vi "Complex Spectrum Averaging.vi"(3 "reset averaging (T)":bool=TRUE, 4 "number of averages":u32=10 min=1, 5 "weighting mode":enum16{"Linear", "Exponential"}(ring), 6 "complex spectrum":cdb[](array[numeric]) format="%.2f") -> (0 "error out":errorcluster, 1 "averages completed":dbl format="%.2f", 2 "averaged complex spectrum":cdb[](array[numeric]) format="%.2f")   [LabVIEW 2017]
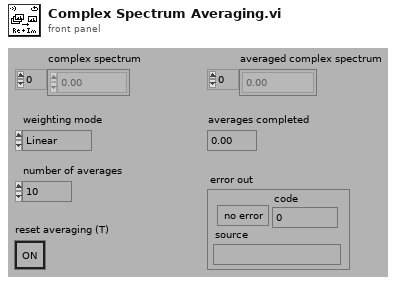
[diagram p1: front panel]
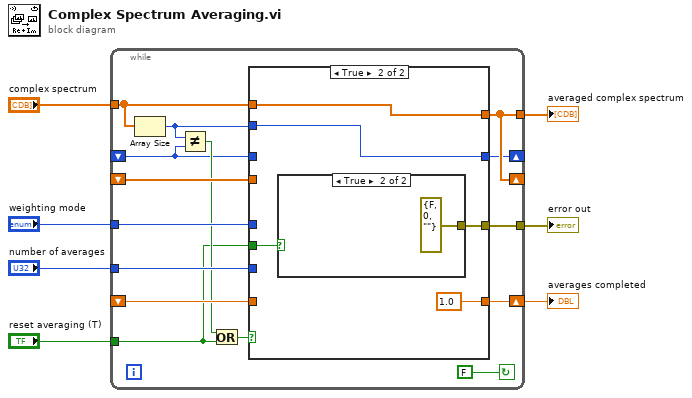
[diagram p0: block diagram]
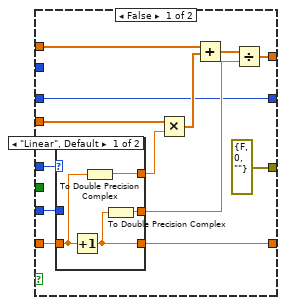
[diagram p2: hidden frame]
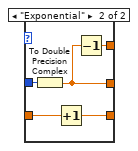
[diagram p3: hidden frame]
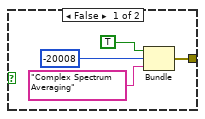
[diagram p4: hidden frame]
diagram:
  n1 = while {
    tunnel: [w11] -> w1
    shift-left: _ -> [w10]
    shift-right: [w15] -> _
    tunnel: "number of averages" -> [w17]
    tunnel: "weighting mode" -> [w18]
    tunnel: "complex spectrum" -> [w16]
    shift-left: _ -> [w20]
    shift-right: [w21] -> w4
    shift-left: _ -> [w19]
    shift-right: [w22] -> _
    tunnel: [w22] -> w5
    tunnel: "reset averaging (T)" -> [w9]
    stop <- FALSE continue-if-true
    n2 = Array Size(array=w16) -> (size(s)=w14:i32)
    n3 = Not Equal?(x=w14, y=w10) -> (x != y?=w12:bool)
    n4 = Or(x=w12, y=w9) -> (x .or. y?=w13:bool)
    n5 = case shown="True" w13 {
      tunnel: [w32 w48] -> w22
      tunnel: [w27 1.0] -> w21
      tunnel: w20 -> [w30 _]
      tunnel: w19 -> [w35 _]
      tunnel: w16 -> [w31 w48]
      tunnel: w18 -> [w28 _]
      tunnel: w17 -> [w25 _]
      tunnel: [w23 w47] -> w15
      tunnel: w14 -> [_ w47]
      tunnel: [errorcluster {FALSE, 0, ""} w46] -> w11
      tunnel: w10 -> [w23 _]
      tunnel: w9 -> [_ w45]
      frame False {
        n6 = case shown="\"Linear\", Default" w28 {
          tunnel: w30 -> [w38 w43]
          tunnel: [w36 w44] -> w27
          tunnel: [w39 w40] -> w29
          tunnel: [w37 w41] -> w26
          tunnel: w25 -> [_ w42]
          frame "Linear", Default {
            n7 = Increment(x=w38) -> (x+1=w36:dbl)
            n8 = To Double Precision Complex(1:w38) -> (0:w39:cdb)
            n9 = To Double Precision Complex(1:w36) -> (0:w37:cdb)
          }
          frame "Exponential" {
            n10 = To Double Precision Complex(1:w42) -> (0:w41:cdb)
            n11 = Increment(x=w43) -> (x+1=w44:dbl)
            n12 = Decrement(x=w41) -> (x-1=w40:cdb)
          }
        }
        n13 = Multiply(x=w35, y=w29) -> (x*y=w34:cdb[])
        n14 = Add(x=w31, y=w34) -> (x+y=w33:cdb[])
        n15 = Divide(x=w33, y=w26) -> (x/y=w32:cdb[])
      }
      frame True {
        n16 = case shown="True" w45 {
          tunnel: [w50 errorcluster {FALSE, 0, ""}] -> w46
          frame False {
            n17 = Bundle(TRUE, -20008, "Complex Spectrum Averaging") -> (w50:errorcluster)  [unwired: 1 in]
          }
          frame True {
          }
        }
      }
    }
  }
  "averaged complex spectrum" <- w5
  "averages completed" <- w4
  "error out" <- w1
